vi "LUCS001RT_GPS_RS232_ReadID_Bytes.vi"(8 "error in":errorcluster, 9 "FPGA VI Reference":refnum<k20>) -> (0 "error out":errorcluster, 1 "FPGA VI Reference Out":refnum<k20>, 2 "ID":u8 format="%02x", 3 "Class":u8 format="%02x", 5 "Length":u16 format="%04x")   [LabVIEW 2024]
uses:
  <vilib>/rvi/interface/nirviMethod/nirviMethod.xnode
  sbRIO-9612/SourceCodeFPGA/LUCS002FPGA_Main.vi
  SourceCode_Host/SourceCode_Host/FPGA Bitfiles/LUCS002h.lvproj_FPGA Target_LUCS002FPGA_Main.vi.lvbit
  <vilib>/FPGAPlugInAG/sbRIO-9612/niLvFpga_ReadFifo_sbRIO-9612.vi
  <vilib>/rvi/errors/niLvFpgaMergeErrorWithErrorCode.vi
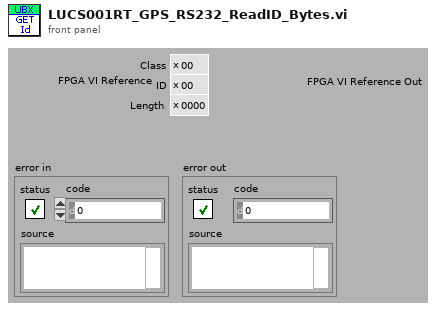
[diagram p1: front panel]
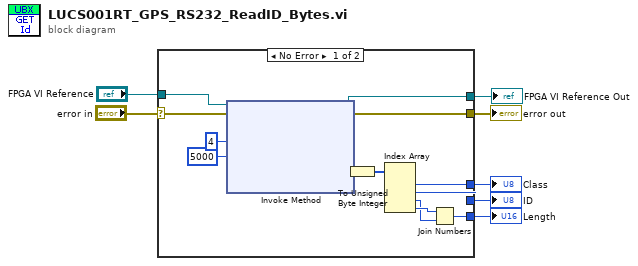
[diagram p0: block diagram]
diagram:
  n1 = case shown="No Error" "error in" {
    selector: "error in" -> [w17 w21]
    tunnel: [w20 _] -> w1
    tunnel: [w19 w21] -> w7
    tunnel: "FPGA VI Reference" -> [w18 _]
    tunnel: [w12 _] -> w5
    tunnel: [w11 _] -> w4
    tunnel: [w8 _] -> w3
    frame No Error {
      n2 = xnode "Invoke Method"("FPGA VI Reference In"=w18, "error in"=w17, "Number of Elements"=u32 4, "Timeout (ms)"=5000) -> ("FPGA VI Reference Out"=w20:refnum<k20>, "error out"=w19:errorcluster, "Data"=w14:void[])  [unwired: 1 out]
      n3 = To Unsigned Byte Integer(number=w14) -> (unsigned 8bit integer=w13:u8[])
      n4 = Index Array(array=w13) -> (element #1=w12:u8, element #2=w11:u8, element #3=w9:u8, element #4=w10:u8)  [unwired: 4 in]
      n5 = Join Numbers(hi=w10, lo=w9) -> ((hi.lo)=w8:u16)
    }
    frame Error {
    }
  }
  "error out" <- w7
  "Class" <- w5
  "ID" <- w4
  "Length" <- w3
  "FPGA VI Reference Out" <- w1
